vi "Teleop.vi"(10 "Match Info":T1={"Autonomous Elapsed Seconds"=0.0, "TeleOp Elapsed Seconds"=0.0, "Disabled Elapsed Seconds"=0.0, "Visited Autonomous"=FALSE, "Visited TeleOp"=FALSE, "Visited Disabled"=FALSE, "Autonomous Settings"={"Autonomous Style"=enum."Independent", "VI Refnum"=refnum}}, 11 "Call Context":T2) -> ()   [LabVIEW 2016]
doc: "This VI is called for each TeleOp packet received from the DS where the robot is not disabled. It is often used to read from the joysticks and update I/O or to update setpoints for timed control loops. It should complete and return within 20 milliseconds or it may miss DS packets."
uses:
  <vilib>/Rock Robotics/WPI/DriverStation/WPI_DriverStationDerivedRobotMode.ctl
  <vilib>/Rock Robotics/WPI/DriverStation/WPI_DriverStationMatch Info.ctl
  <vilib>/Rock Robotics/WPI/Solenoid/WPI_SolenoidValue.ctl
  <vilib>/Rock Robotics/WPI/ThirdParty/CanMotor/TalonSRX/WPI_CANTalonSRX_APIControlMode.ctl
  <vilib>/Rock Robotics/WPI/Utilities/WPI_GetSetVariantRefNum.vi
  <vilib>/Rock Robotics/WPI/Solenoid/WPI_SolenoidSetEnum.vi
  <vilib>/Rock Robotics/Network Tables/NT Read Boolean.vi
  <vilib>/Rock Robotics/Network Tables/NT Read Number.vi
  <vilib>/Rock Robotics/Network Tables/NT Write Boolean.vi
panel:
  in  "gearDegree":dbl
  out "Shooter Target":dbl
  out "Degree Save":dbl
  in  "turntwo":dbl
  in  "degrrees":dbl
  out "Sample Slider 0":dbl(slide) scale=0.0..5.0
  out "Sample Boolean 1":bool
  out "Sample Boolean 0":bool
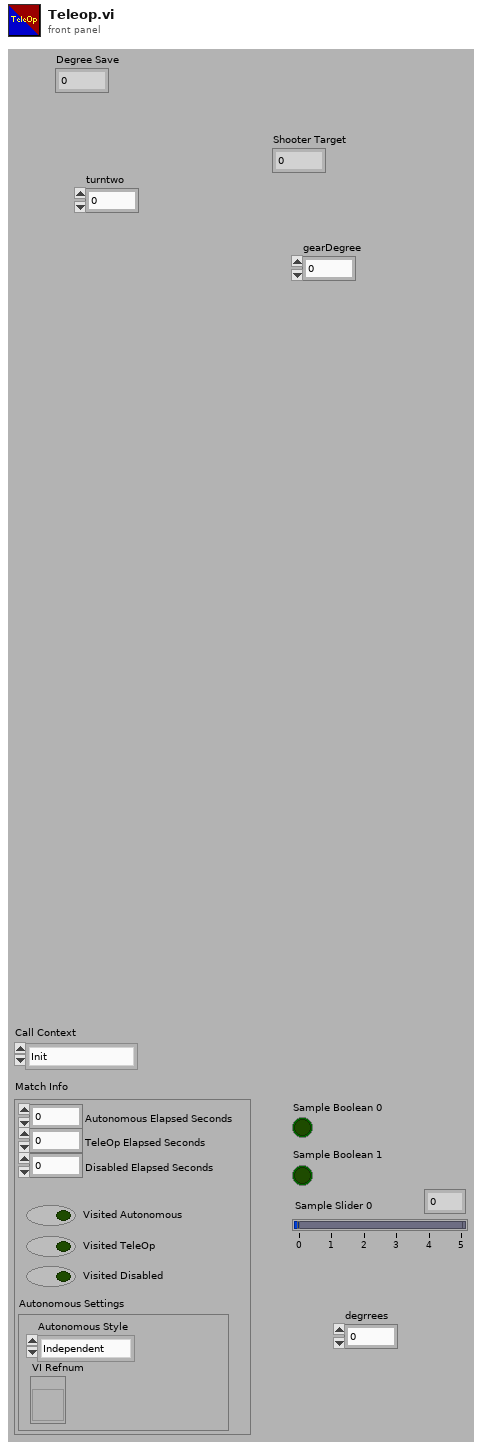
[diagram p1: front panel]
types:
  T1 = typedef "WPI_DriverStationMatch Info.ctl" = cluster{"Autonomous Elapsed Seconds":dbl, "TeleOp Elapsed Seconds":dbl, "Disabled Elapsed Seconds":dbl, "Visited Autonomous":bool, "Visited TeleOp":bool, "Visited Disabled":bool, "Autonomous Settings":cluster{"Autonomous Style":enum16{"Iterative", "Independent"}, "VI Refnum":refnum<vi>}}
  T2 = typedef "WPI_DriverStationDerivedRobotMode.ctl" = enum16{"Init", "Execute", "Stop"}
  T3 = typedef "WPI_SolenoidValue.ctl" = enum16{"Off", "On", "Forward", "Reverse"}
  T4 = typedef "WPI_JoystickDevRef.ctl" = cluster{"Device":T5}
  T5 = typedef "WPI_JoystickDeviceEnum.ctl" = enum16{"USB 0", "USB 1", "USB 2", "USB 3", "USB 4", "USB 5"}
  T6 = cluster{"Buttons[0]":bool, "Buttons[1]":bool, "Buttons[2]":bool, "Buttons[3]":bool, "Buttons[4]":bool, "Buttons[5]":bool, "Buttons[6]":bool, "Buttons[7]":bool, "Buttons[8]":bool}
  T7 = cluster{"Axes[0]":dbl, "Axes[1]":dbl, "Axes[2]":dbl, "Axes[3]":dbl, "Axes[4]":dbl, "Axes[5]":dbl, "Axes[6]":dbl, "Axes[7]":dbl, "Axes[8]":dbl}
  T8 = typedef "WPI_MotorControlDeviceRef.ctl" = cluster{"DeviceStatus":errorcluster, "Type":T9, "PWM":cluster{"PWM Channel":T10, "DeadBand":T11}, "CAN":cluster{"Device Number":u8, "SetOutput VI Ref":variant, "GetOutput VI Ref":variant, "Enable VI Ref":variant, "Disable VI Ref":variant, "Data":variant}, "Invert":bool}
  T9 = typedef "WPI_MotorControlType.ctl" = enum16{"PWM", "CAN"}
  T10 = typedef "FPGA_DIOPWMChannel.ctl" = enum8{"PWM 0", "PWM 1", "PWM 2", "PWM 3", "PWM 4", "PWM 5", "PWM 6", "PWM 7", "PWM 8", "PWM 9", "PWM MXP 0", "PWM MXP 1", "PWM MXP 2", "PWM MXP 3", "PWM MXP 4", "PWM MXP 5", "PWM MXP 6", "PWM MXP 7", "PWM MXP 8", "PWM MXP 9", "Invalid"}
  T11 = typedef "WPI_PWMDeadband.ctl" = cluster{"Name":string, "maxPositivePwm":i32, "minPositivePwm":i32, "centerPwm":i32, "maxNegativePwm":i32, "minNegativePwm":i32, "angularRange":u16}
  T12 = typedef "WPI_SolenoidDevRef.ctl" = cluster{"DevStatus":errorcluster, "Pneumatics Control Module":u8, "Forward Solenoid Channel":T13, "Reverse Solenoid Channel":T13}
  T13 = typedef "WPI_SolenoidChannel.ctl" = enum8{"Solenoid 0", "Solenoid 1", "Solenoid 2", "Solenoid 3", "Solenoid 4", "Solenoid 5", "Solenoid 6", "Solenoid 7", "Invalid"}
  T14 = typedef "WPI_CANTalonSRX_APIControlMode.ctl" = enum8{"Percent VBus", "Speed", "Position", "Slave", "Unchanged / Invalid", "Voltage Compensation", "Current", "Motion Profile", "Motion Magic"}
  T15 = typedef "WPI_SwitchDevRef.ctl" = cluster{"DevStatus":errorcluster, "DIO Channel":T16, "CntIndex":T17, "Normally Closed":bool}
  T16 = typedef "FPGA_DIOChannel.ctl" = enum8{"DIO 0", "DIO 1", "DIO 2", "DIO 3", "DIO 4", "DIO 5", "DIO 6", "DIO 7", "DIO 8", "DIO 9", "DIO MXP 0", "DIO MXP 1", "DIO MXP 2", "DIO MXP 3", "DIO MXP 4", "DIO MXP 5", "DIO MXP 6", "DIO MXP 7", "DIO MXP 8", "DIO MXP 9", "DIO MXP 10", "DIO MXP 11", "DIO MXP 12", "DIO MXP 13", "DIO MXP 14", "DIO MXP 15", "SPI Port CS1", "SPI Port CS2", "SPI Port CS3", "SPI Port MISO", "SPI Port MOSI", "Invalid"}
  T17 = typedef "FPGA_CounterCtrSystemIndex.ctl" = enum8{"Ctr 0", "Ctr 1", "Ctr 2", "Ctr 3", "Ctr 4", "Ctr 5", "Ctr 6", "Ctr 7", "Invalid"}
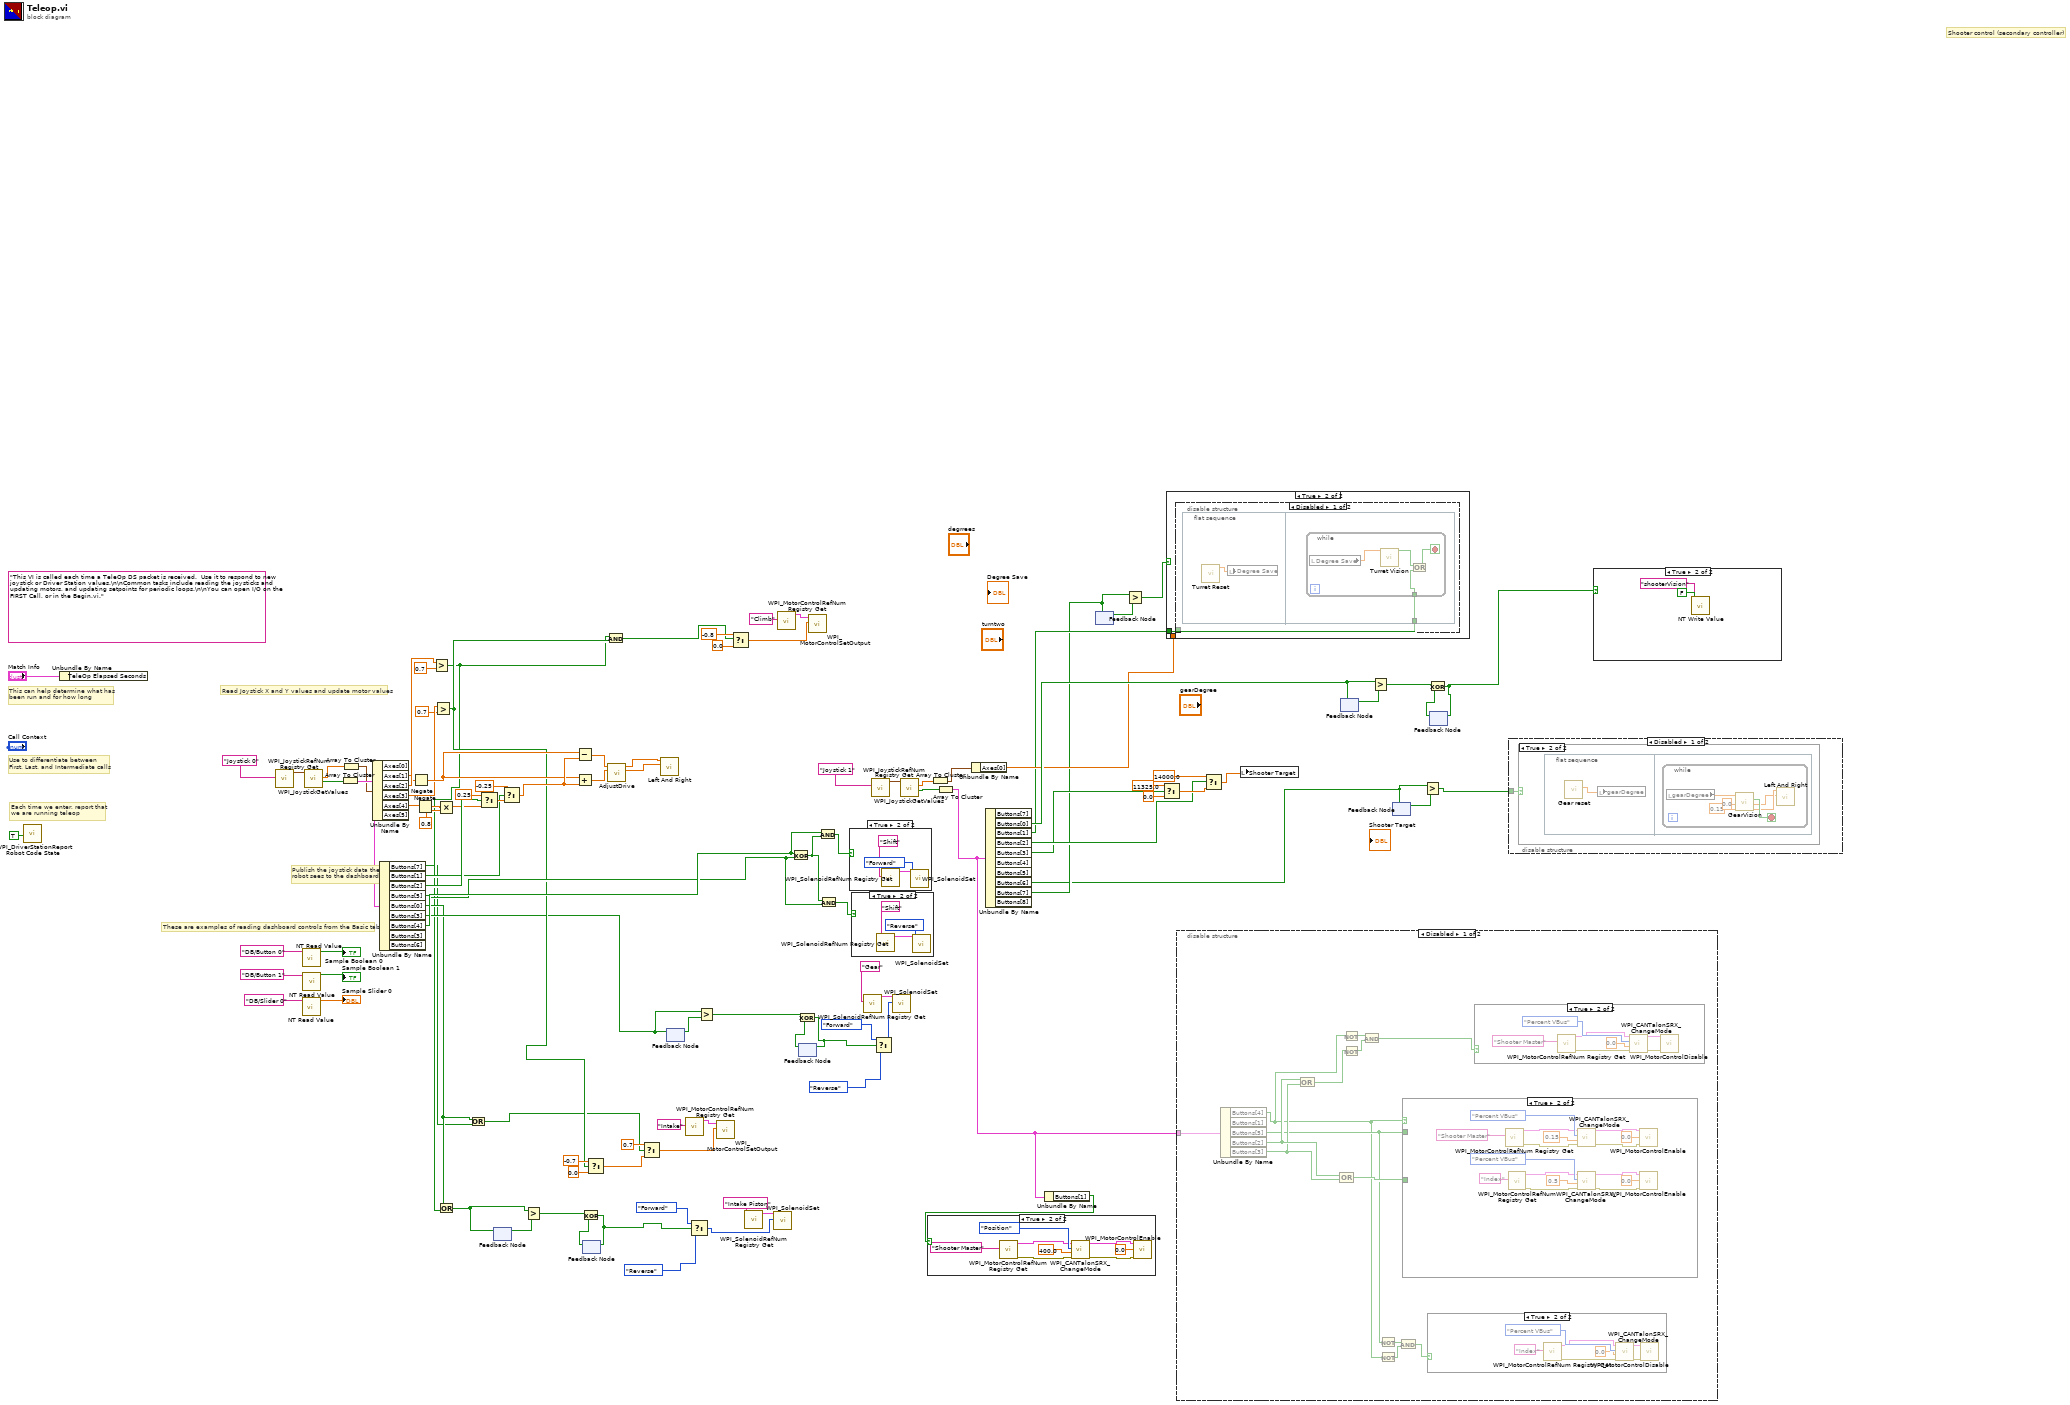
[diagram p0: block diagram]
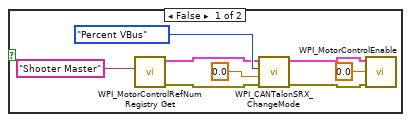
[diagram p2: hidden frame]
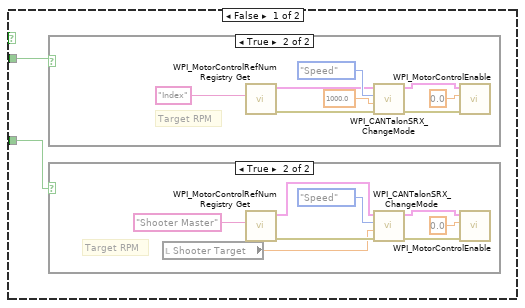
[diagram p3: hidden frame]
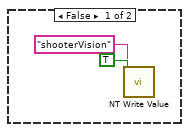
[diagram p11: hidden frame]
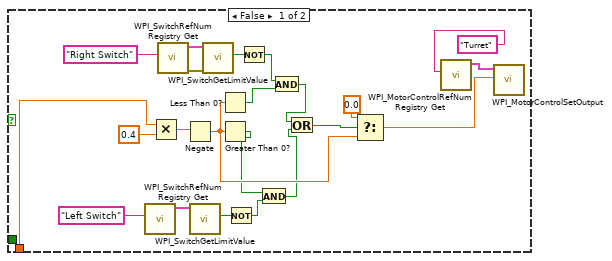
[diagram p12: hidden frame]
diagram:
  (unwired) "This VI is called each time a TeleOp DS packet is received.  Use it to respond to new joystick or Driver Station values.\n\nCommon tasks include reading the joysticks and updating motors, and updating setpoints for periodic loops.\n\nYou can open I/O on the FIRST Call, or in the Begin.vi."
  # "Shooter control (secondary controller)"
  # "These are examples of reading dashboard controls from the Basic tab"
  # "Publish the joystick data the\nrobot sees to the dashboard"
  # "Each time we enter, report that\nwe are running teleop"
  # "Use to differentiate between\nFirst, Last, and Intermediate calls"
  # "This can help determine what has\nbeen run and for how long"
  # "Read Joystick X and Y values and update motor values"
  n1 = call <vilib>:"WPI_DriverStationReport Robot Code State.vi"("TeleOp"=TRUE ("Autonomous")) -> ()  [unwired: 10 in, 1 out]
  n2 = Unbundle By Name("Match Info") -> ()  [unwired: 1 out]
  n3 = call <vilib>:"WPI_JoystickRefNum Registry Get.vi"("refnum name"="Joystick 0") -> ("JoystickDevRef"=w102:T4)  [unwired: 1 in, 9 out]
  n4 = call-poly <vilib>:"NT Read Value.vi"("Name"="DB/Button 0" ("refnum name")) -> ("Boolean"=→"Sample Boolean 0":bool)  [unwired: 9 in, 1 out]
  n5 = call-poly <vilib>:"NT Read Value.vi"("Name"="DB/Slider 0" ("refnum name")) -> ("Numeric"=→"Sample Slider 0":dbl)  [unwired: 9 in, 1 out]
  n6 = call-poly <vilib>:"NT Read Value.vi"("Name"="DB/Button 1" ("refnum name")) -> ("Boolean"=→"Sample Boolean 1":bool)  [unwired: 9 in, 1 out]
  n7 = call <vilib>:"WPI_JoystickGetValues.vi"("JoystickDevRef"=w102) -> ("Buttons"=w94:bool[], "Axes"=w92:dbl[])  [unwired: 6 in, 3 out]
  n8 = Array To Cluster(array=w94) -> (cluster=w93:T6)
  n9 = Array To Cluster(array=w92) -> (cluster=w91:T7)
  n10 = Unbundle By Name(w91) -> ("Axes[1]"=w44:dbl, "Axes[2]"=w76:dbl, "Axes[3]"=w42:dbl, "Axes[4]"=w59:dbl)  [unwired: 2 out]
  n11 = Unbundle By Name(w93) -> ("Buttons[7]"=w25:bool, "Buttons[1]"=w67:bool, "Buttons[2]"=w70:bool, "Buttons[5]"=w61:bool, "Buttons[0]"=w27:bool, "Buttons[3]"=w30:bool, "Buttons[4]"=w62:bool)  [unwired: 2 out]
  n12 = Negate(x=w44) -> (-x=w43:dbl)
  n13 = Negate(x=w59) -> (-x=w58:dbl)
  n14 = Greater?(x=w76, y=0.7) -> (0:w26:bool)
  n15 = Greater?(x=w42, y=0.7) -> (0:w38:bool)
  n16 = Multiply(x=w58, y=0.8) -> (x*y=w63:dbl)
  n17 = Or(x=w27, y=w26) -> (x .or. y?=w29:bool)
  n18 = Or(x=w27, y=w25) -> (x .or. y?=w28:bool)
  n19 = Select(t=0.25, s=w70, f=w63) -> (s? t:f=w69:dbl)
  n20 = feedback #1() -> (w85:bool)  [unwired: 1 in]
  n21 = feedback-in #1(w29) -> ()
  n22 = Select(t=-0.25, s=w67, f=w69) -> (s? t:f=w65:dbl)
  n23 = Greater?(x=w29, y=w85) -> (0:w84:bool)
  n24 = Subtract(x=w43, y=w65) -> (x-y=w72:dbl)
  n25 = Add(x=w43, y=w65) -> (x+y=w71:dbl)
  n26 = feedback #2() -> (w83:bool)  [unwired: 1 in]
  n27 = Exclusive Or(1:w83, 2:w84) -> (0:w32:bool)
  n28 = feedback-in #2(w32) -> ()
  n29 = Select(t=-0.7, s=w38, f=0.0) -> (s? t:f=w37:dbl)
  n30 = And(x=w26, y=w38) -> (x .and. y?=w60:bool)
  n31 = call "AdjustDrive.vi"("Right In"=w71, "Left In"=w72) -> ("Right Out"=w24:dbl, "Left Out"=w23:dbl)  [unwired: 8 in]
  n32 = Select(t=0.7, s=w28, f=w37) -> (s? t:f=w45:dbl)
  n33 = call "Left And Right.vi"("Right"=w24, "Left"=w23) -> ()  [unwired: 10 in]
  n34 = feedback #3() -> (w49:bool)  [unwired: 1 in]
  n35 = feedback-in #3(w30) -> ()
  n36 = call <vilib>:"WPI_MotorControlRefNum Registry Get.vi"("refnum name"="Intake") -> ("MotorControlDevRef"=w47:T8)  [unwired: 9 in, 1 out]
  n37 = Select(t=WPI_SolenoidValue."Forward", s=w32, f=WPI_SolenoidValue."Reverse" ("Value")) -> (s? t:f=w31:T3)
  n38 = Greater?(x=w30, y=w49) -> (0:w57:bool)
  n39 = call <vilib>:"WPI_MotorControlSetOutput.vi"("Output"=w45, "MotorControlDevRef"=w47) -> ()  [unwired: 7 in, 3 out]
  n40 = Select(t=-0.8, s=w60, f=0.0) -> (s? t:f=w86:dbl)
  n41 = call <vilib>:"WPI_SolenoidRefNum Registry Get.vi"("refnum name"="Intake Piston") -> ("SolenoidDevRef"=w35:T12)  [unwired: 9 in, 1 out]
  n42 = call-poly <vilib>:"WPI_SolenoidSet.vi"("Value"=w31, "SolenoidDevRef"=w35) -> ()  [unwired: 8 in, 2 out]
  n43 = call <vilib>:"WPI_MotorControlRefNum Registry Get.vi"("refnum name"="Climb") -> ("MotorControlDevRef"=w90:T8)  [unwired: 9 in, 1 out]
  n44 = Exclusive Or(1:w61, 2:w62) -> (0:w75:bool)
  n45 = feedback #4() -> (w56:bool)  [unwired: 1 in]
  n46 = Exclusive Or(1:w56, 2:w57) -> (0:w50:bool)
  n47 = feedback-in #4(w50) -> ()
  n48 = call <vilib>:"WPI_MotorControlSetOutput.vi"("Output"=w86, "MotorControlDevRef"=w90) -> ()  [unwired: 7 in, 3 out]
  n49 = And(x=w62, y=w75) -> (x .and. y?=w73:bool)
  n50 = And(x=w75, y=w61) -> (x .and. y?=w74:bool)
  n51 = case shown="True" w73 {
    frame False {
    }
    frame True {
      n52 = call <vilib>:"WPI_SolenoidRefNum Registry Get.vi"("refnum name"="Shift") -> ("SolenoidDevRef"=w106:T12)  [unwired: 9 in, 1 out]
      n53 = call-poly <vilib>:"WPI_SolenoidSet.vi"("Value"=WPI_SolenoidValue."Forward", "SolenoidDevRef"=w106) -> ()  [unwired: 8 in, 2 out]
    }
  }
  n54 = case shown="True" w74 {
    frame False {
    }
    frame True {
      n55 = call <vilib>:"WPI_SolenoidRefNum Registry Get.vi"("refnum name"="Shift") -> ("SolenoidDevRef"=w109:T12)  [unwired: 9 in, 1 out]
      n56 = call-poly <vilib>:"WPI_SolenoidSet.vi"("Value"=WPI_SolenoidValue."Reverse", "SolenoidDevRef"=w109) -> ()  [unwired: 8 in, 2 out]
    }
  }
  n57 = call <vilib>:"WPI_SolenoidRefNum Registry Get.vi"("refnum name"="Gear") -> ("SolenoidDevRef"=w54:T12)  [unwired: 9 in, 1 out]
  n58 = call <vilib>:"WPI_JoystickRefNum Registry Get.vi"("refnum name"="Joystick 1") -> ("JoystickDevRef"=w81:T4)  [unwired: 1 in, 9 out]
  n59 = Select(t=WPI_SolenoidValue."Forward", s=w50, f=WPI_SolenoidValue."Reverse" ("Value")) -> (s? t:f=w51:T3)
  n60 = call-poly <vilib>:"WPI_SolenoidSet.vi"("Value"=w51, "SolenoidDevRef"=w54) -> ()  [unwired: 8 in, 2 out]
  n61 = call <vilib>:"WPI_JoystickGetValues.vi"("JoystickDevRef"=w81) -> ("Buttons"=w82:bool[], "Axes"=w79:dbl[])  [unwired: 6 in, 3 out]
  n62 = Array To Cluster(array=w79) -> (cluster=w78:T7)
  n63 = Array To Cluster(array=w82) -> (cluster=w2:T6)
  n64 = Unbundle By Name(w78) -> ("Axes[0]"=w10:dbl)
  n65 = Unbundle By Name(w2) -> ("Buttons[0]"=w13:bool, "Buttons[1]"=w9:bool, "Buttons[2]"=w14:bool, "Buttons[3]"=w12:bool, "Buttons[6]"=w4:bool, "Buttons[7]"=w6:bool)  [unwired: 4 out]
  n66 = Unbundle By Name(w2) -> ("Buttons[1]"=w1:bool)
  n67 = case shown="True" w1 {
    frame False {
      n68 = call <vilib>:"WPI_MotorControlRefNum Registry Get.vi"("refnum name"="Shooter Master") -> ("error out"=w114:errorcluster, "MotorControlDevRef"=w113:T8)  [unwired: 9 in]
      n69 = call <vilib>:"WPI_CANTalonSRX_ChangeMode.vi"("error in (no error)"=w114, "Output"=0.0, "Control Mode"=WPI_CANTalonSRX_APIControlMode."Percent VBus", "CAN Talon SRX Ref"=w113) -> ("error out"=w118:errorcluster, "CAN Talon SRX Ref"=w117:T8)  [unwired: 6 in]
      n70 = call <vilib>:"WPI_MotorControlEnable.vi"("error in (no error)"=w118, "Encoder Initial Position"=0.0, "CAN MotorDevRef"=w117) -> ()  [unwired: 7 in, 2 out]
    }
    frame True {
      n71 = call <vilib>:"WPI_MotorControlRefNum Registry Get.vi"("refnum name"="Shooter Master") -> ("error out"=w122:errorcluster, "MotorControlDevRef"=w121:T8)  [unwired: 9 in]
      n72 = call <vilib>:"WPI_CANTalonSRX_ChangeMode.vi"("error in (no error)"=w122, "Output"=400.0, "Control Mode"=WPI_CANTalonSRX_APIControlMode."Position", "CAN Talon SRX Ref"=w121) -> ("error out"=w126:errorcluster, "CAN Talon SRX Ref"=w125:T8)  [unwired: 6 in]
      n73 = call <vilib>:"WPI_MotorControlEnable.vi"("error in (no error)"=w126, "Encoder Initial Position"=0.0, "CAN MotorDevRef"=w125) -> ()  [unwired: 7 in, 2 out]
    }
  }
  n74 = feedback #5() -> (w8:bool)  [unwired: 1 in]
  n75 = feedback-in #5(w6) -> ()
  n76 = Greater?(x=w6, y=w8) -> (0:w7:bool)
  n77 = Select(t=11325.0, s=w12, f=0.0) -> (s? t:f=w22:dbl)
  n78 = case shown="True" w7 {
    tunnel: w10 -> [w127 _]
    tunnel: w9 -> [_ w149]
    frame False {
      n79 = call <vilib>:"WPI_SwitchRefNum Registry Get.vi"("refnum name"="Left Switch") -> ("SwitchDevRef"=w132:T15)  [unwired: 9 in, 1 out]
      n80 = Multiply(x=w127, y=0.4) -> (x*y=w142:dbl)
      n81 = call <vilib>:"WPI_SwitchRefNum Registry Get.vi"("refnum name"="Right Switch") -> ("error out"=w137:errorcluster, "SwitchDevRef"=w138:T15)  [unwired: 9 in]
      n82 = Negate(x=w142) -> (-x=w146:dbl)
      n83 = call <vilib>:"WPI_SwitchGetLimitValue.vi"("SwitchDevRef"=w132) -> ("Switch Pressed"=w134:bool)  [unwired: 8 in, 2 out]
      n84 = call <vilib>:"WPI_SwitchGetLimitValue.vi"("error in (no error)"=w137, "SwitchDevRef"=w138) -> ("Switch Pressed"=w140:bool)  [unwired: 7 in, 2 out]
      n85 = Less Than 0?(x=w146) -> (x < 0?=w128:bool)
      n86 = Greater Than 0?(x=w146) -> (x > 0?=w129:bool)
      n87 = Not(x=w134) -> (.not. x?=w131:bool)
      n88 = Not(x=w140) -> (.not. x?=w136:bool)
      n89 = And(x=w129, y=w131) -> (x .and. y?=w130:bool)
      n90 = And(x=w136, y=w128) -> (x .and. y?=w135:bool)
      n91 = Or(x=w135, y=w130) -> (x .or. y?=w148:bool)
      n92 = Select(t=0.0, s=w148, f=w146) -> (s? t:f=w144:dbl)
      n93 = call <vilib>:"WPI_MotorControlRefNum Registry Get.vi"("refnum name"="Turret") -> ("MotorControlDevRef"=w145:T8)  [unwired: 9 in, 1 out]
      n94 = call <vilib>:"WPI_MotorControlSetOutput.vi"("Output"=w144, "MotorControlDevRef"=w145) -> ()  [unwired: 7 in, 3 out]
    }
    frame True {
      n95 = disable-structure shown="Disabled" {
        disable-tunnel: w149 -> [w150 _]
        frame Disabled {
          n96 = flat-sequence {
            tunnel: w150 -> [w152]
            frame #0 {
              n97 = call "Turret Reset.vi"() -> ("Numeric"=w151:dbl)  [unwired: 11 in]
              n98 = local write "Degree Save"(w151) -> ()
            }
            frame #1 {
              n99 = while {
                tunnel: w152 -> [w154]
                stop <- w156 stop-if-true
                n100 = local read "Degree Save"() -> (w153:dbl)
                n101 = call "Turret Vision.vi"("Degree Save"=w153) -> ("Boolean"=w155:bool)  [unwired: 10 in]
                n102 = Or(x=w155, y=w154) -> (x .or. y?=w156:bool)
              }
            }
          }
        }
        frame Enabled {
        }
      }
    }
  }
  n103 = disable-structure shown="Disabled" {
    disable-tunnel: w2 -> [w169 _]
    frame Disabled {
      n104 = Unbundle By Name(w169) -> ("Buttons[4]"=w157:bool, "Buttons[5]"=w158:bool, "Buttons[2]"=w161:bool, "Buttons[3]"=w160:bool)  [unwired: 1 out]
      n105 = Compound Arithmetic op=OR(w161, w160) -> (w159:bool)
      n106 = Compound Arithmetic op=OR(w161, w160) -> (w162:bool)
      n107 = Not(x=w157) -> (.not. x?=w165:bool)
      n108 = Not(x=w159) -> (.not. x?=w164:bool)
      n109 = And(x=w165, y=w164) -> (x .and. y?=w163:bool)
      n110 = Not(x=w158) -> (.not. x?=w167:bool)
      n111 = Not(x=w157) -> (.not. x?=w166:bool)
      n112 = And(x=w167, y=w166) -> (x .and. y?=w168:bool)
      n113 = case shown="True" w157 {
        tunnel: w158 -> [w171 _]
        tunnel: w162 -> [w170 _]
        frame False {
          n114 = case shown="True" w171 {
            frame False {
            }
            frame True {
              # "Target RPM"
              n115 = call <vilib>:"WPI_MotorControlRefNum Registry Get.vi"("refnum name"="Index") -> ("error out"=w183:errorcluster, "MotorControlDevRef"=w182:T8)  [unwired: 9 in]
              n116 = call <vilib>:"WPI_CANTalonSRX_ChangeMode.vi"("error in (no error)"=w183, "Output"=1000.0, "Control Mode"=WPI_CANTalonSRX_APIControlMode."Speed", "CAN Talon SRX Ref"=w182) -> ("error out"=w187:errorcluster, "CAN Talon SRX Ref"=w186:T8)  [unwired: 6 in]
              n117 = call <vilib>:"WPI_MotorControlEnable.vi"("error in (no error)"=w187, "Encoder Initial Position"=0.0, "CAN MotorDevRef"=w186) -> ()  [unwired: 7 in, 2 out]
            }
          }
          n118 = case shown="True" w170 {
            frame False {
            }
            frame True {
              # "Target RPM"
              n119 = local read "Shooter Target"() -> (w172:dbl)
              n120 = call <vilib>:"WPI_MotorControlRefNum Registry Get.vi"("refnum name"="Shooter Master") -> ("error out"=w174:errorcluster, "MotorControlDevRef"=w175:T8)  [unwired: 9 in]
              n121 = call <vilib>:"WPI_CANTalonSRX_ChangeMode.vi"("error in (no error)"=w174, "Output"=w172, "Control Mode"=WPI_CANTalonSRX_APIControlMode."Speed", "CAN Talon SRX Ref"=w175) -> ("error out"=w177:errorcluster, "CAN Talon SRX Ref"=w176:T8)  [unwired: 6 in]
              n122 = call <vilib>:"WPI_MotorControlEnable.vi"("error in (no error)"=w177, "Encoder Initial Position"=0.0, "CAN MotorDevRef"=w176) -> ()  [unwired: 7 in, 2 out]
            }
          }
        }
        frame True {
          n123 = call <vilib>:"WPI_MotorControlRefNum Registry Get.vi"("refnum name"="Shooter Master") -> ("error out"=w199:errorcluster, "MotorControlDevRef"=w198:T8)  [unwired: 9 in]
          n124 = call <vilib>:"WPI_MotorControlRefNum Registry Get.vi"("refnum name"="Index") -> ("error out"=w191:errorcluster, "MotorControlDevRef"=w190:T8)  [unwired: 9 in]
          n125 = call <vilib>:"WPI_CANTalonSRX_ChangeMode.vi"("error in (no error)"=w199, "Output"=0.15, "Control Mode"=WPI_CANTalonSRX_APIControlMode."Percent VBus", "CAN Talon SRX Ref"=w198) -> ("error out"=w203:errorcluster, "CAN Talon SRX Ref"=w202:T8)  [unwired: 6 in]
          n126 = call <vilib>:"WPI_CANTalonSRX_ChangeMode.vi"("error in (no error)"=w191, "Output"=0.5, "Control Mode"=WPI_CANTalonSRX_APIControlMode."Percent VBus", "CAN Talon SRX Ref"=w190) -> ("error out"=w195:errorcluster, "CAN Talon SRX Ref"=w194:T8)  [unwired: 6 in]
          n127 = call <vilib>:"WPI_MotorControlEnable.vi"("error in (no error)"=w203, "Encoder Initial Position"=0.0, "CAN MotorDevRef"=w202) -> ()  [unwired: 7 in, 2 out]
          n128 = call <vilib>:"WPI_MotorControlEnable.vi"("error in (no error)"=w195, "Encoder Initial Position"=0.0, "CAN MotorDevRef"=w194) -> ()  [unwired: 7 in, 2 out]
        }
      }
      n129 = case shown="True" w168 {
        frame False {
        }
        frame True {
          n130 = call <vilib>:"WPI_MotorControlRefNum Registry Get.vi"("refnum name"="Index") -> ("error out"=w209:errorcluster, "MotorControlDevRef"=w208:T8)  [unwired: 9 in]
          n131 = call <vilib>:"WPI_CANTalonSRX_ChangeMode.vi"("error in (no error)"=w209, "Output"=0.0, "Control Mode"=WPI_CANTalonSRX_APIControlMode."Percent VBus", "CAN Talon SRX Ref"=w208) -> ("error out"=w205:errorcluster, "CAN Talon SRX Ref"=w204:T8)  [unwired: 6 in]
          n132 = call <vilib>:"WPI_MotorControlDisable.vi"("error in (no error)"=w205, "MotorControlDevRef"=w204) -> ()  [unwired: 8 in, 2 out]
        }
      }
      n133 = case shown="True" w163 {
        frame False {
        }
        frame True {
          n134 = call <vilib>:"WPI_MotorControlRefNum Registry Get.vi"("refnum name"="Shooter Master") -> ("error out"=w216:errorcluster, "MotorControlDevRef"=w215:T8)  [unwired: 9 in]
          n135 = call <vilib>:"WPI_CANTalonSRX_ChangeMode.vi"("error in (no error)"=w216, "Output"=0.0, "Control Mode"=WPI_CANTalonSRX_APIControlMode."Percent VBus", "CAN Talon SRX Ref"=w215) -> ("error out"=w212:errorcluster, "CAN Talon SRX Ref"=w211:T8)  [unwired: 6 in]
          n136 = call <vilib>:"WPI_MotorControlDisable.vi"("error in (no error)"=w212, "MotorControlDevRef"=w211) -> ()  [unwired: 8 in, 2 out]
        }
      }
    }
    frame Enabled {
    }
  }
  n137 = Select(t=14000.0, s=w14, f=w22) -> (s? t:f=w19:dbl)
  n138 = local write "Shooter Target"(w19) -> ()
  n139 = feedback #6() -> (w18:bool)  [unwired: 1 in]
  n140 = feedback-in #6(w13) -> ()
  n141 = Greater?(x=w13, y=w18) -> (0:w17:bool)
  n142 = feedback #7() -> (w5:bool)  [unwired: 1 in]
  n143 = feedback-in #7(w4) -> ()
  n144 = Greater?(x=w4, y=w5) -> (0:w3:bool)
  n145 = feedback #8() -> (w16:bool)  [unwired: 1 in]
  n146 = Exclusive Or(1:w16, 2:w17) -> (0:w15:bool)
  n147 = feedback-in #8(w15) -> ()
  n148 = disable-structure shown="Disabled" {
    disable-tunnel: w3 -> [w218 _]
    frame Disabled {
      n149 = case shown="True" w218 {
        frame False {
        }
        frame True {
          n150 = flat-sequence {
            frame #0 {
              n151 = call "Gear reset.vi"() -> ("GearDegrees"=w219:dbl)  [unwired: 11 in]
              n152 = local write "gearDegree"(w219) -> ()
            }
            frame #1 {
              n153 = while {
                stop <- w222 stop-if-true
                n154 = local read "gearDegree"() -> (w225:dbl)
                n155 = call "GearVision.vi"("Turn"=0.15, "Forward"=0.0, "gearDegrees"=w225) -> ("gearVisionLeft"=w221:dbl, "gearVisionRight"=w220:dbl, "Kill"=w222:bool)  [unwired: 6 in]
                n156 = call "Left And Right.vi"("Right"=w220, "Left"=w221) -> ()  [unwired: 10 in]
              }
            }
          }
        }
      }
    }
    frame Enabled {
    }
  }
  n157 = case shown="True" w15 {
    frame False {
      n158 = call-poly <vilib>:"NT Write Value.vi"("Boolean"=TRUE, "Name"="shooterVision") -> ()  [unwired: 9 in, 1 out]
    }
    frame True {
      n159 = call-poly <vilib>:"NT Write Value.vi"("Boolean"=FALSE, "Name"="shooterVision") -> ()  [unwired: 9 in, 1 out]
    }
  }
